vi "Config Move Buttons.vi"(8 "error in (no error)":errorcluster, 11 "Configuration in":refnum<class "Configuration.lvclass">) -> (0 "error out":errorcluster, 3 "Configuration out":refnum<class "Configuration.lvclass">)   [LabVIEW 2016, in "Hardware.lvlib" / "VacuumLine.lvlib" / "VacuumLine Configuration.lvclass"]
uses:
  <userlib>/Common Components/Hardware/Abstract System/VacuumLine/VacuumLine Config/VacuumLine Configuration.lvclass
  <userlib>/Configuration Dialog Actor/Configuration.lvclass
  <userlib>/Common Components/Hardware/Abstract System/VacuumLine/VacuumLine/Button Config Cluster.ctl
  C:/Program Files (x86)/National Instruments/LabVIEW 2016/user.lib/Configuration Dialog Actor/Configuration.lvclass
  C:/Program Files (x86)/National Instruments/LabVIEW 2016/vi.lib/ActorFramework/Actor/Actor.lvclass
  <userlib>/Common Components/Hardware/Abstract System/VacuumLine/VacuumLine Config/VacuumLine Configuration.lvclass/VacuumLine Configuration.ctl
  <userlib>/Common Components/Hardware/Abstract System/VacuumLine/VacuumLine/VacuumLine.lvclass/VacuumLine.ctl
  <vilib>/ActorFramework/Actor/Actor.lvclass/Actor.ctl
  <userlib>/Common Components/Hardware/Abstract System/VacuumLine/VacuumLine/Read Array of Move Button Configurations.vi
  <userlib>/Common Components/Hardware/Abstract System/VacuumLine/VacuumLine/Write Array of Move Button Configurations.vi
  <vilib>/ActorFramework/Actor/Actor.lvclass
  <userlib>/Common Components/Hardware/Abstract System/VacuumLine/VacuumLine/VacuumLine.lvclass
panel:
  in  "Array of Button Configurations":T1[](array[typedef]) {"Target pos" format="%#_f mm"}
  in  "Revert":bool
  in  "Apply":bool
  # "Enabled?"
  # "Text on button"
  # "Target pos"
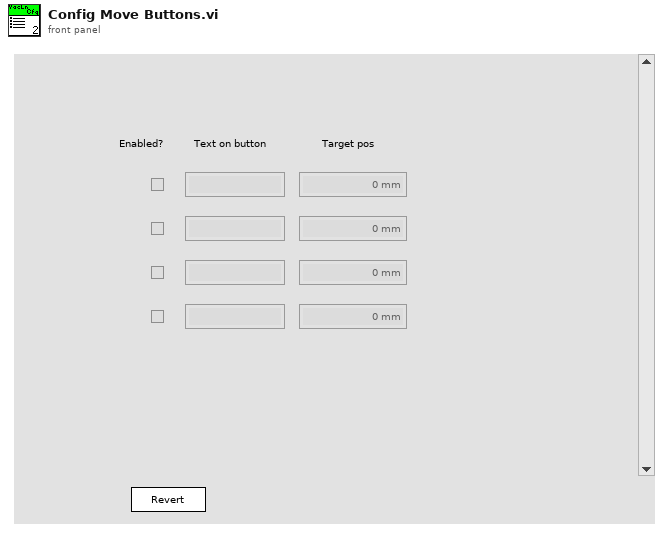
[diagram p1: front panel]
types:
  T1 = typedef "Hardware.lvlib/VacuumLine.lvlib/VacuumLine.lvclass/Button Config Cluster.ctl" = cluster{"Enabled?":bool, "Text on button":string, "Target pos":dbl}
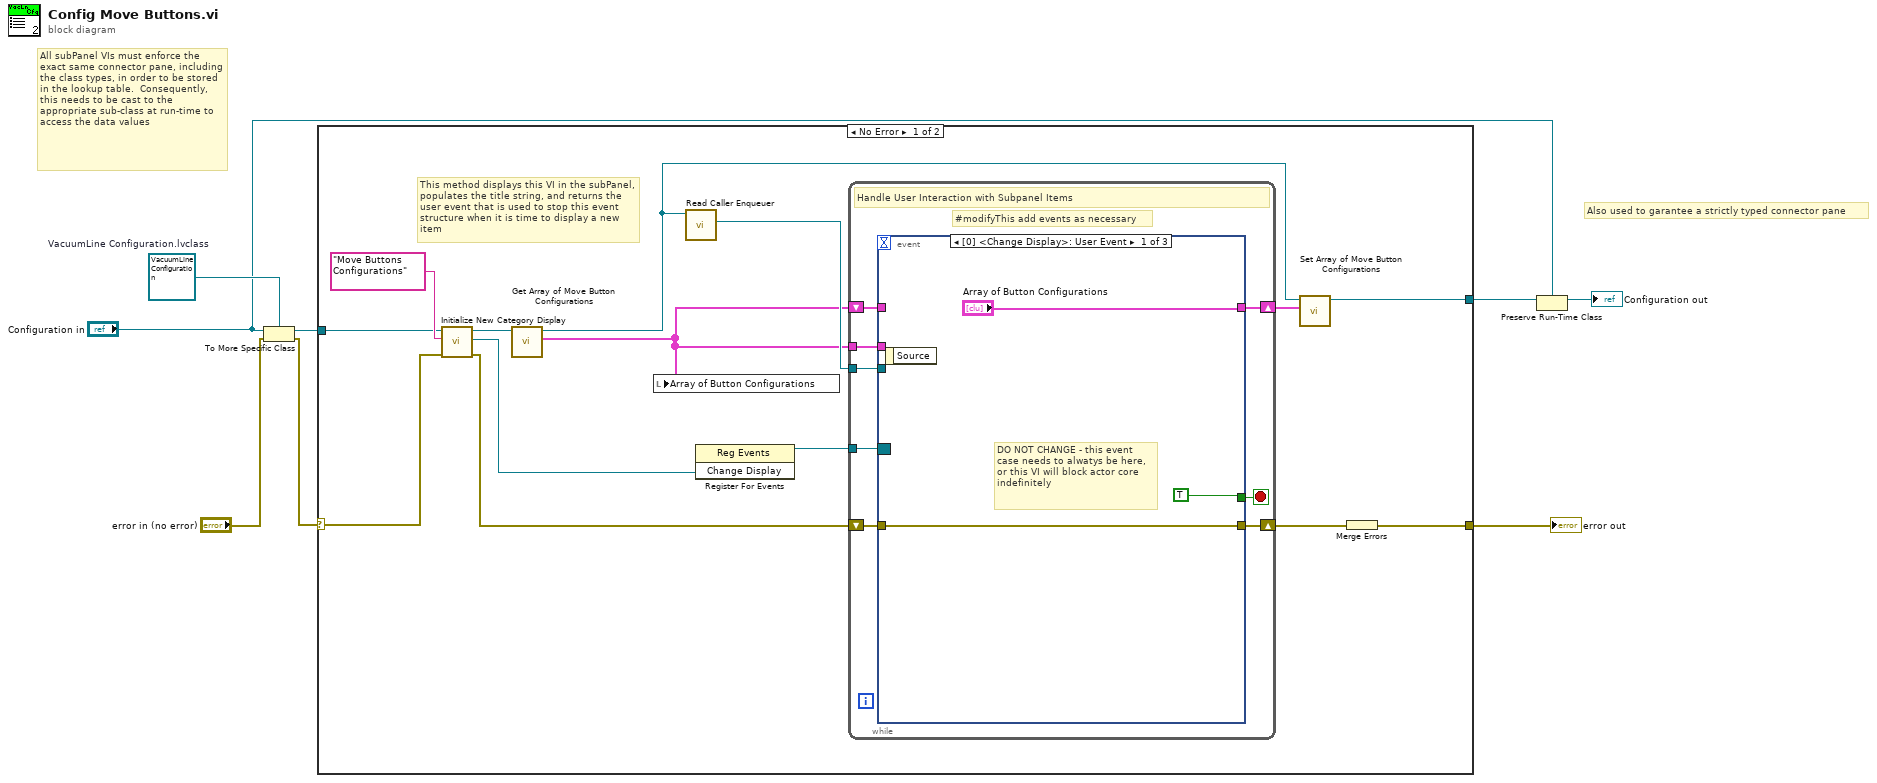
[diagram p0: block diagram]
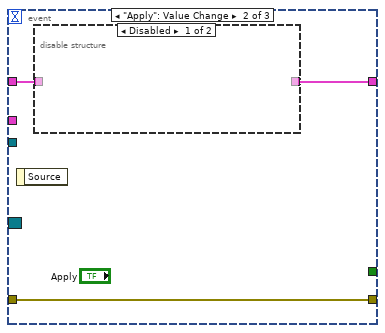
[diagram p2: hidden frame]
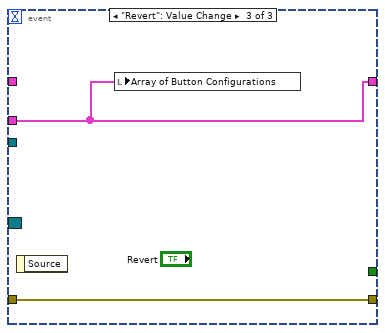
[diagram p4: hidden frame]
diagram:
  w5 = refnum<class "VacuumLine Configuration.lvclass"> refnum  # VacuumLine Configuration.lvclass
  # "Also used to garantee a strictly typed connector pane"
  # "All subPanel VIs must enforce the exact same connector pane, including the class types, in order to be stored in the lookup table.  Consequently, this needs to be cast to the appropriate sub-class at run-time to access the data values"
  n1 = To More Specific Class(target class=w5, reference="Configuration in", error in="error in (no error)") -> (specific class reference=w6:refnum<class "VacuumLine Configuration.lvclass">, error out=w1:errorcluster)
  n2 = case shown="No Error" w1 {
    selector: w1 -> [w16 w40]
    tunnel: w6 -> [w10 w41]
    tunnel: [w12 w41] -> w8
    tunnel: [w22 w40] -> w7
    frame No Error {
      # "This method displays this VI in the subPanel, populates the title string, and returns the user event that is used to stop this event structure when it is time to display a new item"
      n3 = call <userlib>:"Initialize New Category Display.vi"("error in (no error)"=w16, "Name to Display"="Move Buttons Configurations", "Configuration in"=w10) -> ("error out"=w17:errorcluster, "Change Display"=w20:refnum<user-event>, "Configuration Out"=w14:refnum<class "VacuumLine Configuration.lvclass">)  [unwired: 6 in]
      n4 = call <userlib>:"Get Array of Move Button Configurations.vi"("VacuumLine Configuration in"=w14) -> ("Array of Move Button Configurations"=w11:T1[], "VacuumLine Configuration out"=w13:refnum<class "VacuumLine Configuration.lvclass">)  [unwired: 8 in, 1 out]
      n5 = local write "Array of Button Configurations"(w11) -> ()
      n6 = call <vilib>:"Read Caller Enqueuer.vi"("Actor"=w13) -> ("Caller Enqueuer"=w15:refnum<class "Message Enqueuer.lvclass">)  [unwired: 10 in]
      n7 = register-events(w20) -> (reference out=w19:refnum<event-registration>)  [unwired: 2 in, 1 out]
      n8 = while {
        tunnel: w19 -> [w29]
        shift-right: [w28] -> w18
        shift-left: w17 -> [w27]
        shift-right: [w25] -> w9
        shift-left: w11 -> [w26]
        tunnel: w11 -> [w24]
        tunnel: w15 -> [w23]
        stop <- w30 stop-if-true
        # "#modifyThis add events as necessary"
        # "Handle User Interaction with Subpanel Items"
        n9 = event shown="[0] <Change Display>: User Event" {
          selector: w29 -> [_ _ _]
          dyn-events: _ -> [_ _ _]
          timeout: _ -> [_ _ _]
          tunnel: [TRUE _ _] -> w30
          tunnel: [w33 w36 w39] -> w28
          tunnel: w27 -> [w33 w36 w39]
          tunnel: w26 -> [_ w34 _]
          tunnel: ["Array of Button Configurations" w35 w38] -> w25
          tunnel: w24 -> [_ _ w38]
          tunnel: w23 -> [_ _ _]
          event User Event {
            # "DO NOT CHANGE - this event case needs to alwatys be here, or this VI will block actor core indefinitely"
            n10 = event-data() -> ()  [unwired: 1 in, 1 out]
          }
          event "Apply": Value Change {
            n11 = event-data() -> ()  [unwired: 1 in, 1 out]
            n12 = disable-structure shown="Disabled" {
              disable-tunnel: [_ w37] -> w35
              disable-tunnel: w34 -> [_ w37]
              frame Disabled {
              }
              frame Enabled {
              }
            }
          }
          event "Revert": Value Change {
            n13 = event-data() -> ()  [unwired: 1 in, 1 out]
            n14 = local write "Array of Button Configurations"(w38) -> ()
          }
        }
      }
      n15 = call <userlib>:"Set Array of Move Button Configurations.vi"("Array of Move Button Configurations"=w9, "VacuumLine Configuration in"=w13) -> ("VacuumLine Configuration out"=w12:refnum<class "VacuumLine Configuration.lvclass">)  [unwired: 8 in, 1 out]
      n16 = Merge Errors(w18) -> (w22:errorcluster)
    }
    frame Error {
    }
  }
  "error out" <- w7
  n17 = Preserve Run-Time Class(object in=w8, 2:"Configuration in") -> (object out=→"Configuration out":refnum<class "Configuration.lvclass">)  [unwired: 1 in, 1 out]
